vi "Keyence.Main.WaitForInit.vi"(11 "idx":i32) -> ()   [LabVIEW 2016]
uses:
  Keyence.Data.Status.State.ctl
  Global/ApplicationGlobal.vi
  LowLevel/Keyence.Global.vi
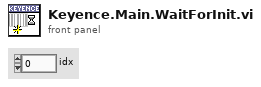
[diagram p1: front panel]
types:
  T1 = typedef "Keyence.Data.Status.State.ctl" = enum16{"First", "Init", "Reset", "Idle", "Scan", "Tune"}
  T2 = typedef "Keyence.Data.Status.ctl" = cluster{"State":T1, "Ref":refnum<k5>, "Bank":u8, "Version":string, "Model":string, "EndTS":timestamp, "ImgPath":path, "Tuned":bool}
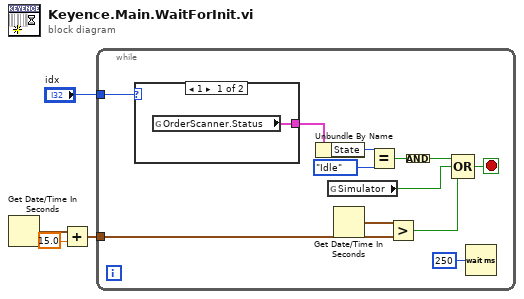
[diagram p0: block diagram]
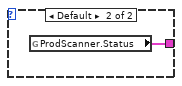
[diagram p2: hidden frame]
diagram:
  n1 = Get Date/Time In Seconds() -> (seconds since 1Jan1904=w4:timestamp)
  n2 = Add(x=w4, y=15.0) -> (x+y=w2:timestamp)
  n3 = while {
    tunnel: w2 -> [w12]
    tunnel: "idx" -> [w6]
    stop <- w8 stop-if-true
    n4 = case shown="1" w6 {
      tunnel: [w17 w18] -> w7
      frame 1 {
        n5 = global read "Keyence.Global.vi" "OrderScanner.Status"() -> (w17:T2)
      }
      frame Default {
        n6 = global read "Keyence.Global.vi" "ProdScanner.Status"() -> (w18:T2)
      }
    }
    n7 = Unbundle By Name(w7) -> ("State"=w16:T1)
    n8 = global read "ApplicationGlobal.vi" "Simulator"() -> (w9:bool)
    n9 = Get Date/Time In Seconds() -> (seconds since 1Jan1904=w11:timestamp)
    n10 = Equal?(x=w16, y=Keyence.Data.Status.State."Idle") -> (x = y?=w15:bool)
    n11 = Greater?(x=w11, y=w12) -> (0:w10:bool)
    n12 = Compound Arithmetic op=AND(w15) -> (w14:bool)
    n13 = Compound Arithmetic op=OR(w14, w9, w10) -> (w8:bool)
    n14 = Wait (ms)(milliseconds to wait=u32 250) -> ()  [unwired: 1 out]
  }
